vi "halfadder (SubVI).vi"(10 "Boolean 2":bool, 11 "Boolean":bool) -> (2 "carry":bool, 3 "sum":bool)   [LabVIEW 2015]
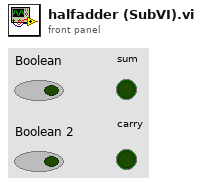
[diagram p1: front panel]
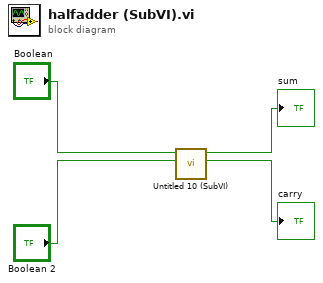
[diagram p0: block diagram]
diagram:
  n1 = call "Untitled 10 (SubVI).vi"("Boolean 2"="Boolean 2", "Boolean"="Boolean") -> ("carry"=→"carry":bool, "sum"=→"sum":bool)  [unwired: 8 in]
